vi "Log User Events.vi"(7 "Log Message":string, 10 "error in (no error)":errorcluster) -> (2 "error out":errorcluster)   [LabVIEW 2020]
uses:
  Database/Controls/DB Options.ctl
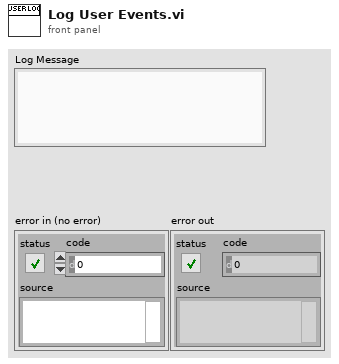
[diagram p1: front panel]
types:
  T1 = enum16{"open", "replace", "create", "open or create", "replace or create", "replace or create with confirmation"}
  T2 = enum32{"invalid app kind", "Development System", "Run Time System", "Student Edition", "Embedded LabVIEW", "Evaluation", "Custom"}
  T3 = typedef "DB Options.ctl" = enum16{"Select", "Execute", "Special Q", "Insert", "Update", "Delete", "Open", "Close"}
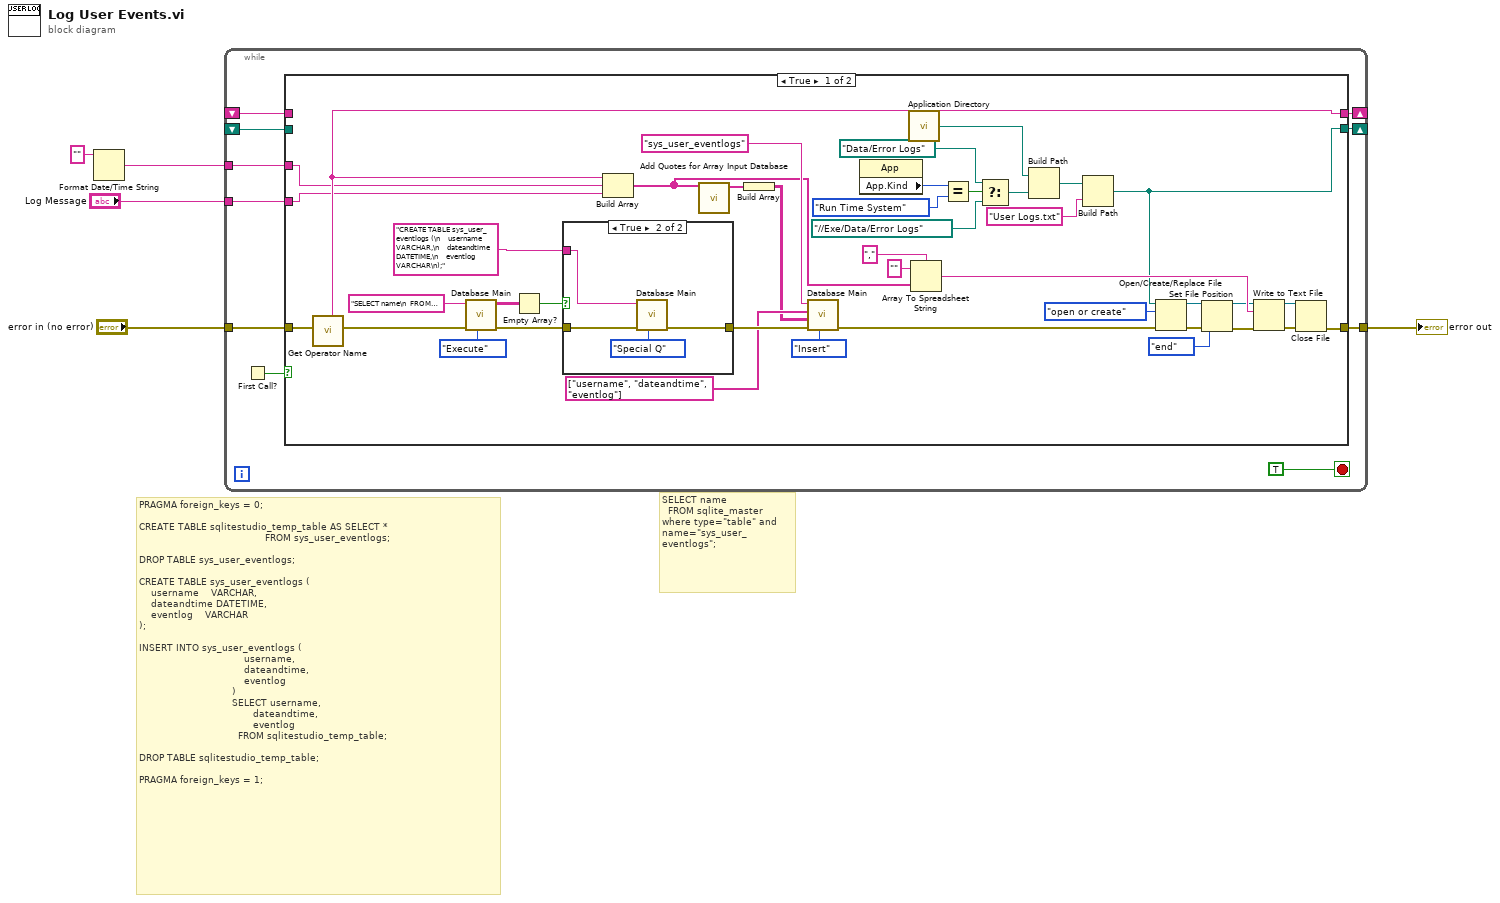
[diagram p0: block diagram]
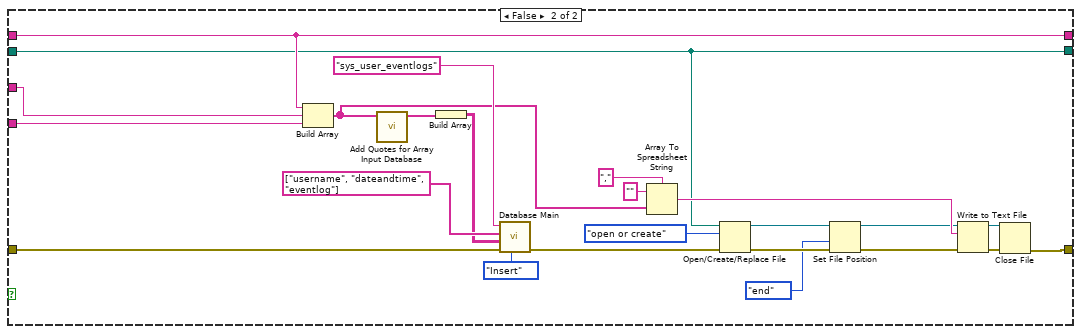
[diagram p3: hidden frame]
diagram:
  # "SELECT name\n  FROM sqlite_master where type=\"table\" and name=\"sys_user_eventlogs\";"
  # "PRAGMA foreign_keys = 0;\n\nCREATE TABLE sqlitestudio_temp_table AS SELECT *\n                                          FROM sys_user_eventlogs;\n\nDROP TABLE sys_user_eventlogs;\n\nCREATE TABLE sys_user_eventlogs (\n    username    VARCHAR,\n    dateandtime DATETIME,\n    eventlog    VARCHAR\n);\n\nINSERT INTO sys_user_eventlogs (\n                                   username,\n                                   dateandtime,\n                                   eventlog\n                               )\n                               SELECT username,\n                                      dateandtime,\n                                      eventlog\n                                 FROM sqlitestudio_temp_table;\n\nDROP TABLE sqlitestudio_temp_table;\n\nPRAGMA foreign_keys = 1;"
  n1 = Format Date/Time String(time format string (%c)="") -> (date/time string=w2:string)  [unwired: 2 in]
  n2 = while {
    tunnel: "error in (no error)" -> [w14]
    tunnel: [w13] -> w4
    shift-right: [w12] -> _
    shift-left: _ -> [w11]
    tunnel: "Log Message" -> [w10]
    tunnel: w2 -> [w9]
    shift-right: [w7] -> _
    shift-left: _ -> [w6]
    stop <- TRUE stop-if-true
    n3 = First Call?() -> (First Call?: T/F=w15:bool)
    n4 = case shown="True" w15 {
      tunnel: w14 -> [w56 w78]
      tunnel: [w23 w70] -> w13
      tunnel: [w46 w79] -> w12
      tunnel: w11 -> [_ w79]
      tunnel: w10 -> [w44 w83]
      tunnel: w9 -> [w45 w84]
      tunnel: [w22 w67] -> w7
      tunnel: w6 -> [_ w67]
      frame True {
        n5 = call "Get Operator Name.vi"("error in (no error)"=w56) -> ("error out"=w54:errorcluster, "Operator Name"=w46:string)  [unwired: 9 in]
        n6 = call "Database Main.vi"("Option"=DB_Options."Execute", "error in (no error)"=w54, "table Name/Query"="SELECT name\n  FROM sqlite_master where type=\"table\" and name=\"sys_user_eventlogs\";\n") -> ("error out"=w50:errorcluster, "Data"=w52:string[][])  [unwired: 6 in, 1 out]
        n7 = Empty Array?(array=w52) -> (empty?=w51:bool)
        n8 = case shown="True" w51 {
          tunnel: w50 -> [w57 w60]
          tunnel: [w57 w59] -> w47
          tunnel: "CREATE TABLE sys_user_eventlogs (\n    username    VARCHAR,\n    dateandtime DATETIME,\n    eventlog    VARCHAR\n);" ("table Name/Query") -> [_ w58]
          frame False {
          }
          frame True {
            n9 = call "Database Main.vi"("Option"=DB_Options."Special Q", "error in (no error)"=w60, "table Name/Query"=w58) -> ("error out"=w59:errorcluster)  [unwired: 6 in, 2 out]
          }
        }
        n10 = Build Array(w46, w45, w44) -> (w30:string[])
        n11 = call "Add Quotes for Array Input Database.vi"("Array Input"=w30) -> ("Array Out"=w21:string[])  [unwired: 10 in]
        n12 = Build Array(w21) -> (w42:string[][])
        n13 = call "Database Main.vi"("Option"=DB_Options."Insert", "error in (no error)"=w47, "Column Values"=w42, "Column Name"=string[] ["username", "dateandtime", "eventlog"], "table Name/Query"="sys_user_eventlogs") -> ("error out"=w27:errorcluster)  [unwired: 4 in, 2 out]
        n14 = property class="App"() -> ("App.Kind"=w40:T2)  [unwired: 2 in, 2 out]
        n15 = call <vilib>:"Application Directory.vi"() -> ("Application Directory"=w37:path)
        n16 = Array To Spreadsheet String(delimiter (Tab)=",", array=w30, 3:"" ("format string")) -> (spreadsheet string=w31:string)
        n17 = Equal?(x=w40, y=T2."Run Time System") -> (x = y?=w38:bool)
        n18 = Select(t=path "Data/Error Logs" ("Application Directory"), s=w38, f=path "../../Exe/Data/Error Logs" ("Application Directory")) -> (s? t:f=w36:path)
        n19 = Build Path(base path=w37, name or relative path=w36) -> (appended path=w33:path)
        n20 = Build Path(base path=w33, name or relative path="User Logs.txt") -> (appended path=w22:path)
        n21 = Open/Create/Replace File(file path (use dialog)=w22, error in=w27, operation (0:open)=T1."open or create") -> (refnum out=w18:refnum<file>, error out=w20:errorcluster)  [unwired: 3 in, 1 out]
        n22 = Set File Position(refnum=w18, from (0:start)=enum16{"start", "end", "current"}."end", error in=w20) -> (refnum out=w17:refnum<file>, error out=w19:errorcluster)  [unwired: 1 in]
        n23 = Write to Text File(file (use dialog)=w17, text=w31, error in=w19) -> (refnum out=w24:refnum<file>, error out=w25:errorcluster)  [unwired: 1 in, 1 out]
        n24 = Close File(refnum=w24, error in=w25) -> (error out=w23:errorcluster)  [unwired: 1 out]
      }
      frame False {
        n25 = Build Array(w79, w84, w83) -> (w69:string[])
        n26 = call "Add Quotes for Array Input Database.vi"("Array Input"=w69) -> ("Array Out"=w68:string[])  [unwired: 10 in]
        n27 = Build Array(w68) -> (w81:string[][])
        n28 = call "Database Main.vi"("Option"=DB_Options."Insert", "error in (no error)"=w78, "Column Values"=w81, "Column Name"=string[] ["username", "dateandtime", "eventlog"], "table Name/Query"="sys_user_eventlogs") -> ("error out"=w71:errorcluster)  [unwired: 4 in, 2 out]
        n29 = Array To Spreadsheet String(delimiter (Tab)=",", array=w69, 3:"" ("format string")) -> (spreadsheet string=w77:string)
        n30 = Open/Create/Replace File(file path (use dialog)=w67, error in=w71, operation (0:open)=T1."open or create") -> (refnum out=w64:refnum<file>, error out=w66:errorcluster)  [unwired: 3 in, 1 out]
        n31 = Set File Position(refnum=w64, from (0:start)=enum16{"start", "end", "current"}."end", error in=w66) -> (refnum out=w63:refnum<file>, error out=w65:errorcluster)  [unwired: 1 in]
        n32 = Write to Text File(file (use dialog)=w63, text=w77, error in=w65) -> (refnum out=w72:refnum<file>, error out=w73:errorcluster)  [unwired: 1 in, 1 out]
        n33 = Close File(refnum=w72, error in=w73) -> (error out=w70:errorcluster)  [unwired: 1 out]
      }
    }
  }
  "error out" <- w4
